vi "Destroy.vi"(8 "error in":errorcluster, 11 "message ref in":refnum<class "CLM_LocalMessage_UserEvent.lvclass">) -> (0 "error out":errorcluster)   [LabVIEW 2013, in "CLM_LocalMessage_UserEvent.lvclass"]
uses:
  CLM_LocalMessage_UserEvent.lvclass
  CLM_LocalMessage_UserEvent.lvclass/CLM_LocalMessage_UserEvent.ctl
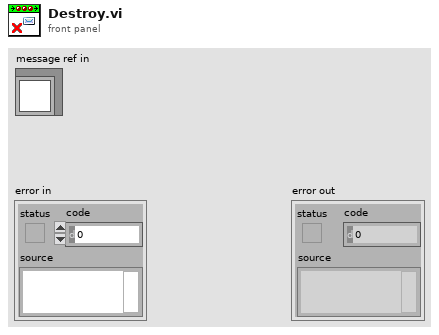
[diagram p1: front panel]
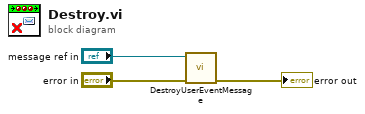
[diagram p0: block diagram]
diagram:
  n1 = call "DestroyUserEventMessage.vi"("error in"="error in", "message ref in"="message ref in") -> ("error out"=→"error out":errorcluster)  [unwired: 9 in]
